vi "ReadEnergy_Ophir.vi"(11 "VISA resource":refnum<visa-resource-name>) -> (0 "error out":errorcluster, 2 "Energy/Power(SI)":dbl)   [LabVIEW 2011]
uses:
  <vilib>/Analysis/NI_AALBase.lvlib
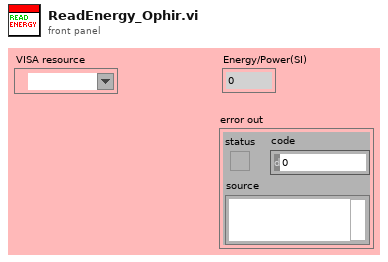
[diagram p1: front panel]
types:
  T1 = enum16{"Initialize", "Write", "Write/Read", "Read", "Clear", "Close"}
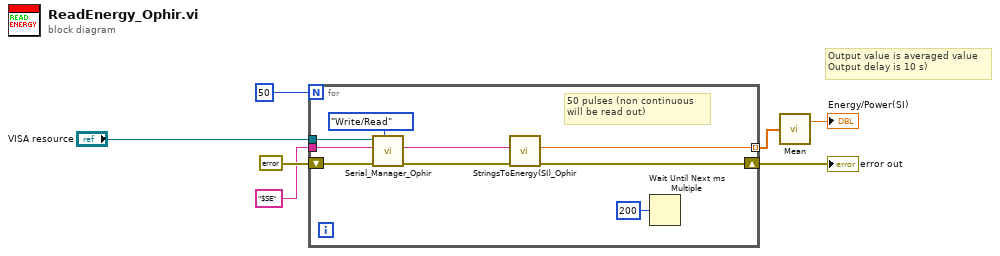
[diagram p0: block diagram]
diagram:
  # "Output value is averaged value\nOutput delay is 10 s)"
  n1 = for {
    N: 50 -> [_]
    tunnel: "VISA resource" -> [w15]
    tunnel: "$SE" ("write buffer") -> [w13]
    shift-right: [w9] -> w7
    shift-left: errorcluster {"status"=FALSE, "code"=0, "source"=""} ("error out") -> [w14]
    tunnel: [w10] -> w2 mode=indexing
    # "50 pulses (non continuous \nwill be read out)"
    n2 = call "Serial_Manager_Ophir.vi"("Job"=T1."Write/Read", "error in"=w14, "write buffer"=w13, "VISA resource"=w15) -> ("error out"=w11:errorcluster, "read buffer"=w12:string)  [unwired: 6 in]
    n3 = call "StringsToEnergy(SI)_Ophir.vi"("error in"=w11, "input string"=w12) -> ("error out"=w9:errorcluster, "Energy/Power(SI)"=w10:dbl)  [unwired: 8 in]
    n4 = Wait Until Next ms Multiple(millisecond multiple=u32 200) -> ()  [unwired: 1 out]
  }
  "error out" <- w7
  n5 = call <vilib>:"Mean.vi"("X"=w2) -> ("mean"=→"Energy/Power(SI)":dbl)  [unwired: 1 out]
